vi "Proper Case.vi"(10 "String in":string) -> (2 "Proper Cased":string)   [LabVIEW 2020, in "Conditum-Tools.lvlib"]
uses:
  Conditum-Tools.lvlib
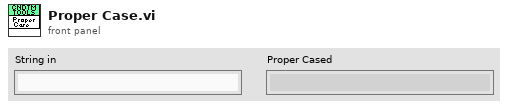
[diagram p1: front panel]
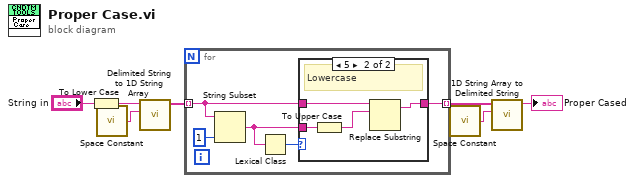
[diagram p0: block diagram]
diagram:
  n1 = To Lower Case(string="String in") -> (all lower case string=w6:string)
  n2 = call <vilib>:"Space Constant.vi"() -> ("String"=w5:string)
  n3 = call <vilib>:"Delimited String to 1D String Array.vi"("delimiter"=w5, "delimited string"=w6) -> ("string array"=w4:string[])  [unwired: 9 in]
  n4 = for {
    tunnel: w4 -> [w10] mode=indexing
    tunnel: [w8] -> w3 mode=indexing
    n5 = String Subset(string=w10, length (rest)=1 ("length (rest)")) -> (substring=w9:string)  [unwired: 1 in]
    n6 = Lexical Class(1:w9) -> (0:w11:i16)
    n7 = case shown="5" w11 {
      tunnel: w10 -> [w13 w16]
      tunnel: w9 -> [_ w17]
      tunnel: [w13 w14] -> w8
      frame Default {
      }
      frame 5 {
        # "Lowercase"
        n8 = To Upper Case(1:w17) -> (0:w15:string)
        n9 = Replace Substring(4:w15, 5:w16) -> (1:w14:string)  [unwired: 2 in, 1 out]
      }
    }
  }
  n10 = call <vilib>:"Space Constant.vi"() -> ("String"=w2:string)
  n11 = call <vilib>:"1D String Array to Delimited String.vi"("delimiter"=w2, "string array"=w3) -> ("delimited string"=→"Proper Cased":string)  [unwired: 9 in]
